vi "Tenscion Analizer.vi"(8 "error in":errorcluster, 11 "Data In":T1) -> (0 "error out":errorcluster, 3 "Data Out":T1)   [LabVIEW 2025]
uses:
  Controls/Wheel_data.ctl
  Controls/Spork plot.ctl
  Controls/Spoke_stats.ctl
  Controls/Spork type.ctl
  Controls/Tension.ctl
  Controls/Tension_Output.ctl
  Controls/Runout.ctl
  Controls/Runout Output.ctl
  Controls/Nippel Turn Direction.ctl
  Controls/Aditional Info.ctl
  <vilib>/Analysis/NI_AALBase.lvlib
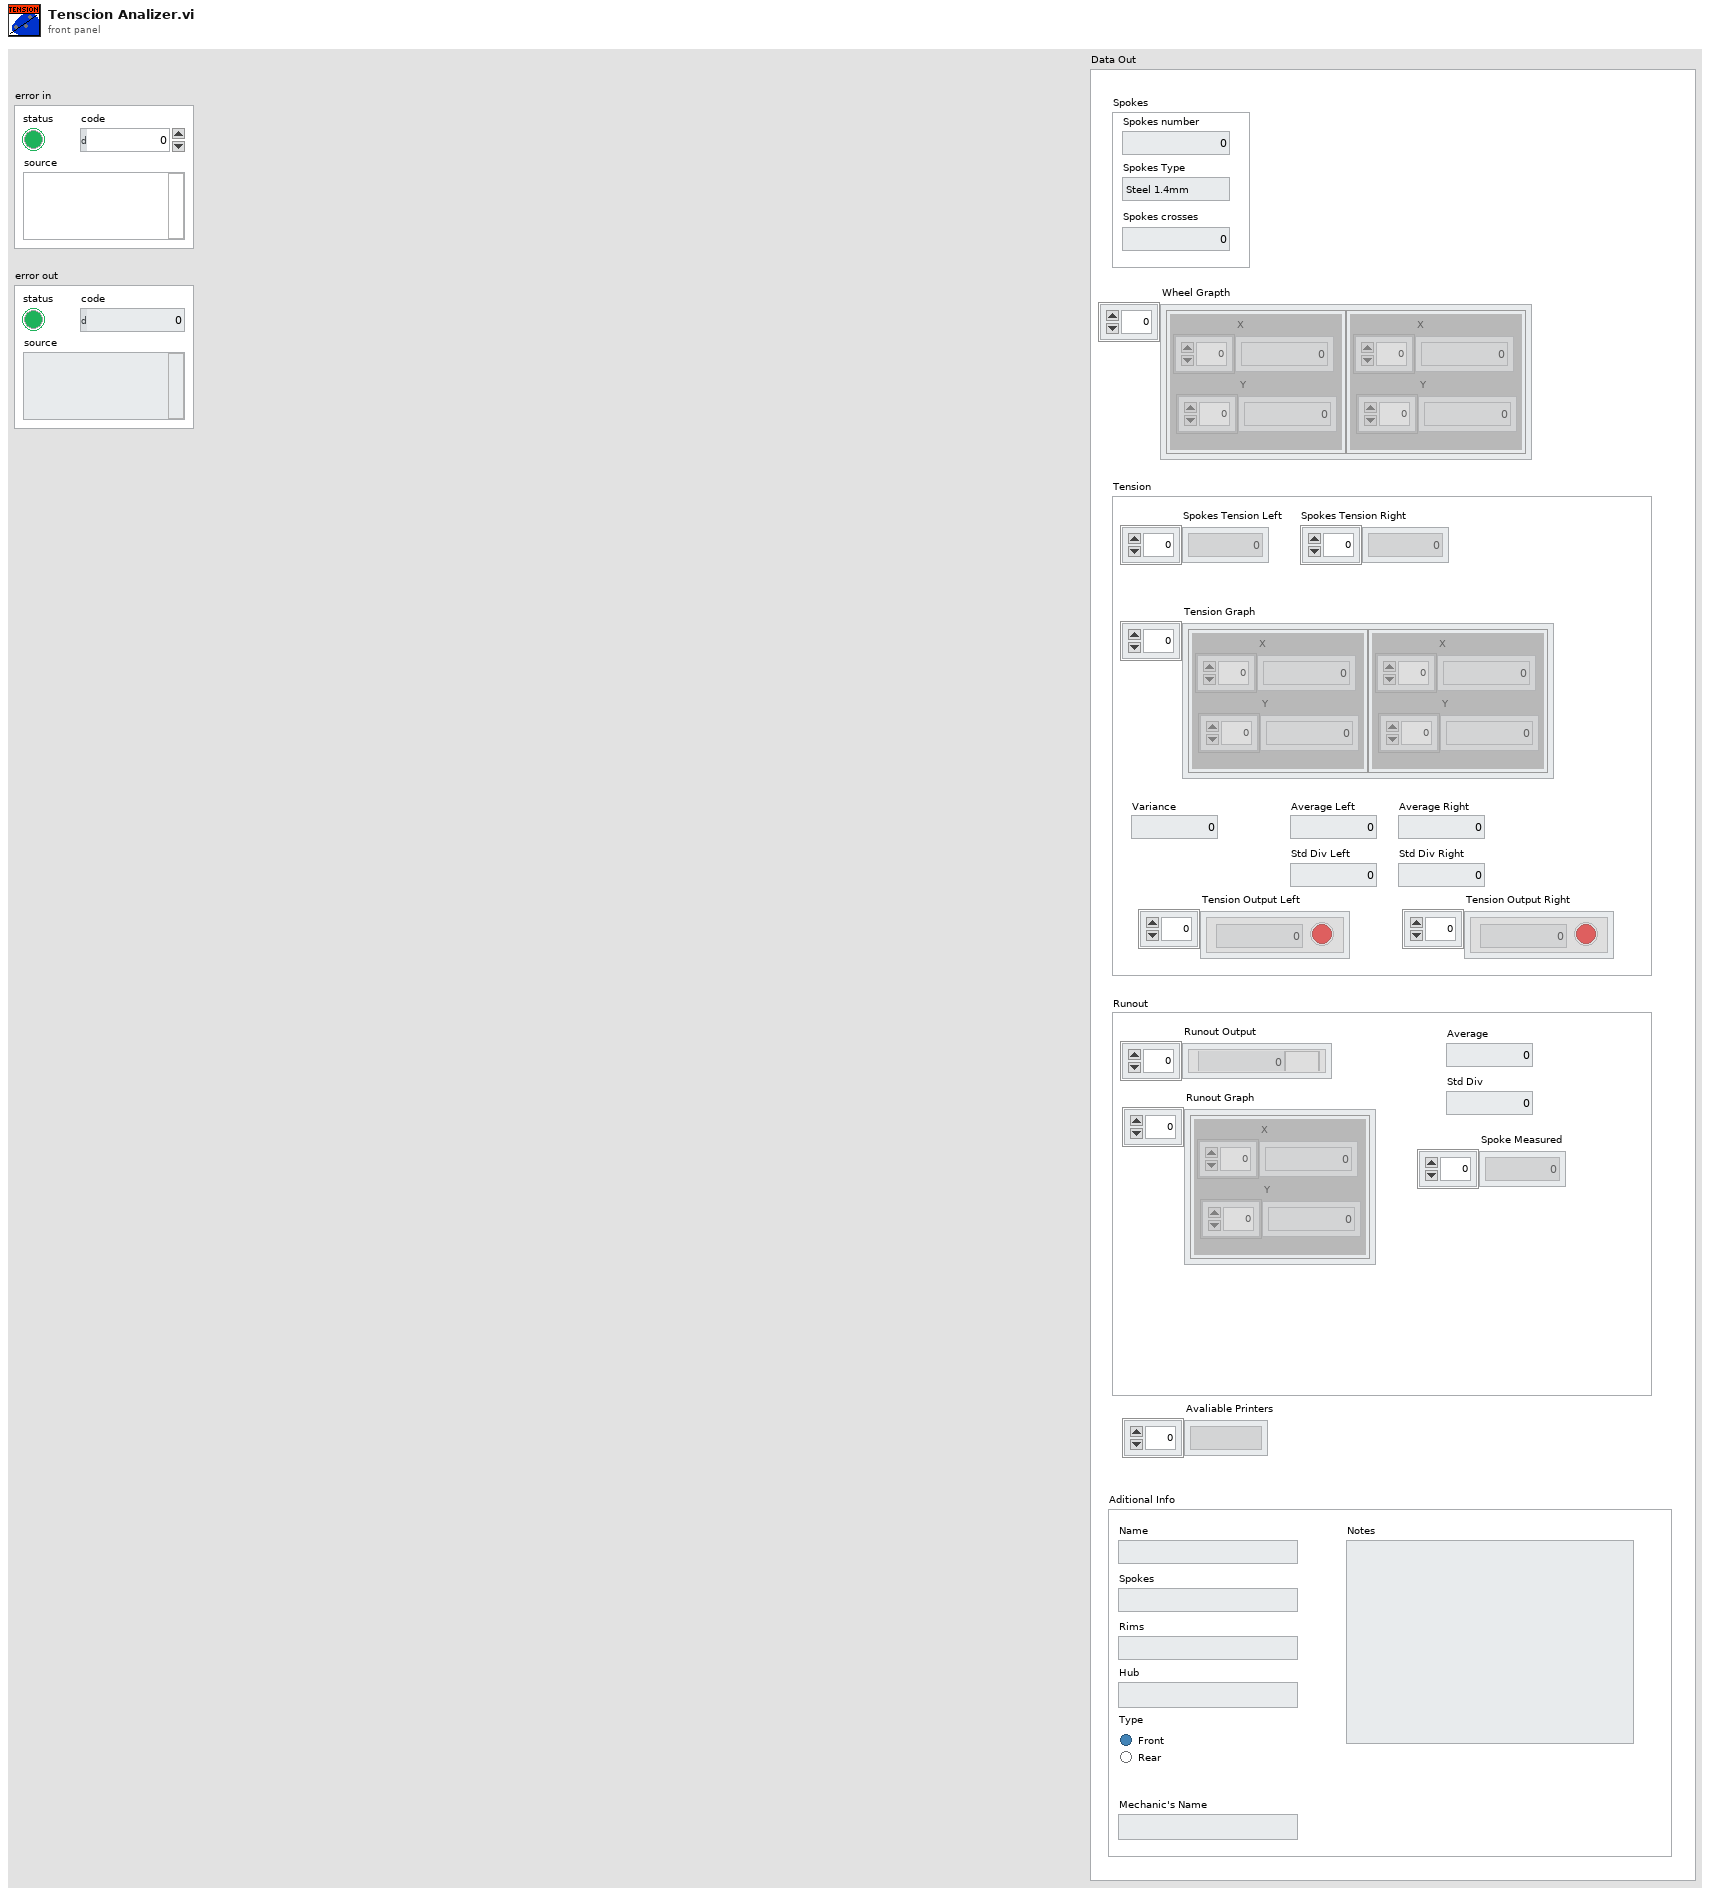
[diagram p1: front panel]
types:
  T1 = typedef "Wheel_data.ctl" = cluster{"Wheel Grapth":T2[], "Spokes":T3, "Tension":T5, "Runout":T7, "Avaliable Printers":string[], "Aditional Info":T10}
  T2 = typedef "Spork plot.ctl" = cluster{"X":dbl[], "Y":dbl[]}
  T3 = typedef "Spoke_stats.ctl" = cluster{"Spokes number":i32, "Spokes crosses":i32, "Spokes Type":T4}
  T4 = typedef "Spork type.ctl" = enum16{"Steel 1.4mm", "Steel 1.5mm", "Steel 1.6mm", "Steel 1.7mm", "Steel 1.8mm", "Steel 2mm", "Steel 2.3mm", "Steel 2.5mm", "Steel 2.6mm", "Aluminum 2.28mm", "Aluminum 2.54mm", "Aluminum 2.8mm", "Aluminum 3.3mm"}
  T5 = typedef "Tension.ctl" = cluster{"Spokes Tension Left":dbl[], "Tension Graph":T2[], "Average Left":dbl, "Variance":dbl, "Std Div Left":dbl, "Average Right":dbl, "Std Div Right":dbl, "Tension Output Left":T6[], "Tension Output Right":T6[], "Spokes Tension Right":dbl[]}
  T6 = typedef "Tension_Output.ctl" = cluster{"Tenction [kgf]":dbl, "Within Limit":bool}
  T7 = typedef "Runout.ctl" = cluster{"Runout Output":T8[], "Runout Graph":T2[], "Average":dbl, "Std Div":dbl, "Spoke Measured":i32[]}
  T8 = typedef "Runout Output.ctl" = cluster{"Value":dbl, "Nippel Direction":T9}
  T9 = typedef "Nippel Turn Direction.ctl" = u16
  T10 = typedef "Aditional Info.ctl" = cluster{"Name":string, "Rims":string, "Hub":string, "Notes":string, "Spokes":string, "Type":enum32{"Item 0", "Item 1"}, "Mechanic's Name":string}
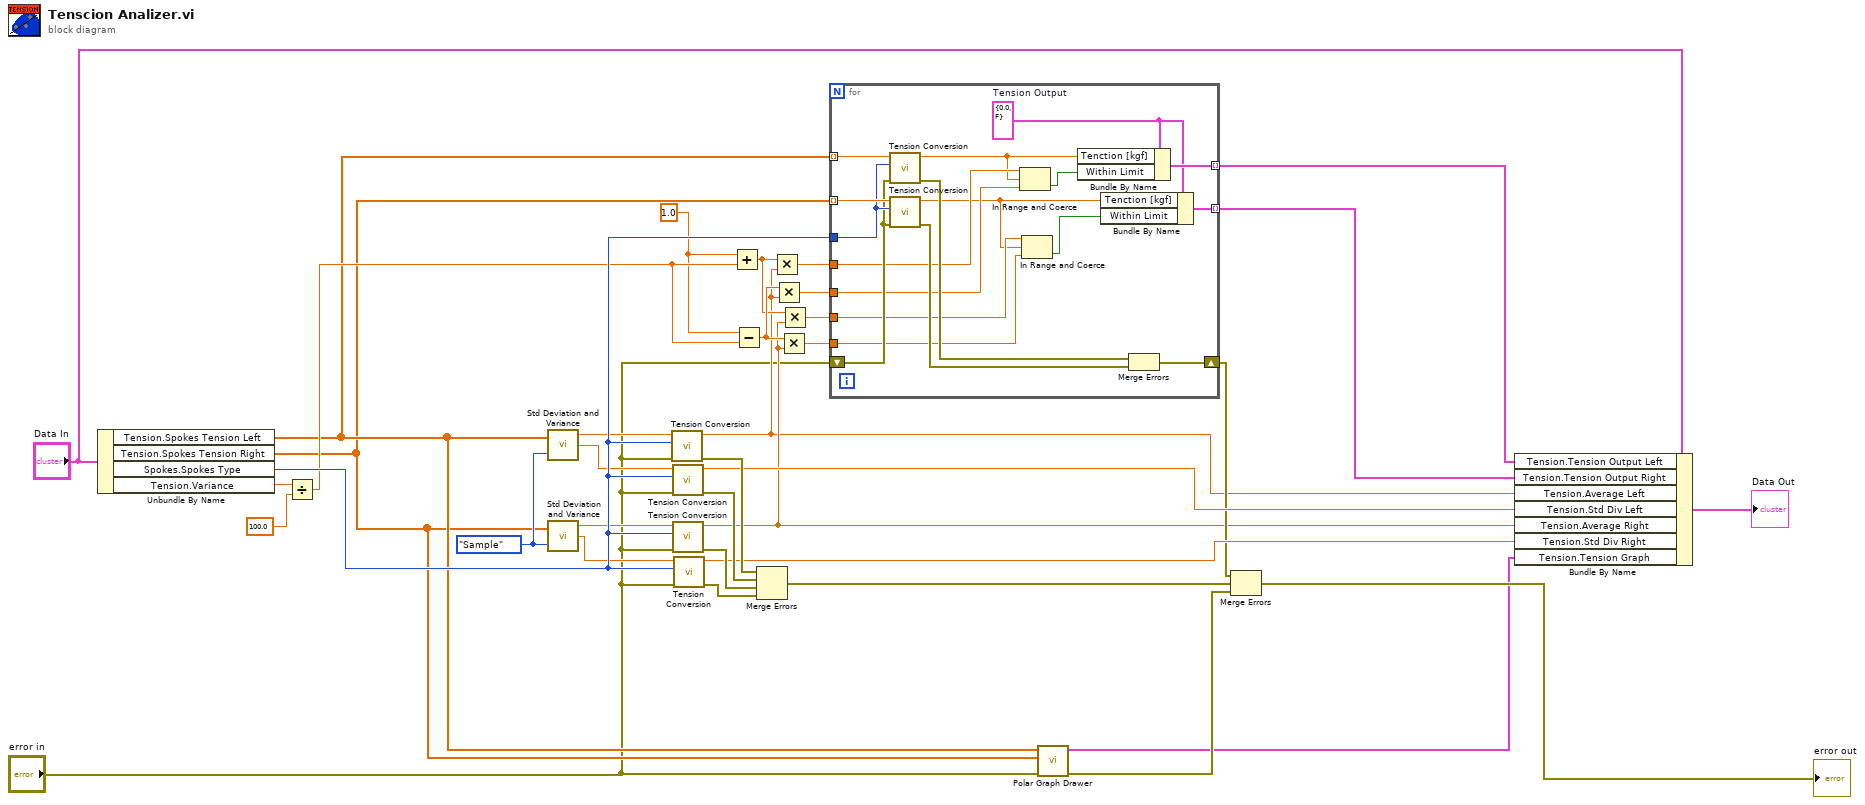
[diagram p0: block diagram]
diagram:
  w22 = 1.0 ("x")
  w7 = enum16{"Sample", "Population"}."Sample" ("Weighting (Sample)")
  n1 = Unbundle By Name("Data In") -> ("Tension.Spokes Tension Left"=w6:dbl[], "Tension.Spokes Tension Right"=w5:dbl[], "Spokes.Spokes Type"=w28:T4, "Tension.Variance"=w25:dbl)
  n2 = Divide(x=w25, y=100.0) -> (x/y=w23:dbl)
  n3 = call <vilib>:"Std Deviation and Variance.vi"("X"=w6, "Weighting (Sample)"=w7) -> ("mean"=w27:dbl, "standard deviation"=w18:dbl)  [unwired: 1 out]
  n4 = call <vilib>:"Std Deviation and Variance.vi"("X"=w5, "Weighting (Sample)"=w7) -> ("mean"=w26:dbl, "standard deviation"=w16:dbl)  [unwired: 1 out]
  n5 = call "Tension Conversion.vi"("error in"="error in", "Spoke Type"=w28, "Tension Input"=w27) -> ("error out"=w31:errorcluster, "Tension [kgf]"=w8:dbl)  [unwired: 6 in, 1 out]
  n6 = call "Tension Conversion.vi"("error in"="error in", "Spoke Type"=w28, "Tension Input"=w18) -> ("error out"=w32:errorcluster, "Tension [kgf]"=w30:dbl)  [unwired: 6 in, 1 out]
  n7 = call "Tension Conversion.vi"("error in"="error in", "Spoke Type"=w28, "Tension Input"=w26) -> ("error out"=w33:errorcluster, "Tension [kgf]"=w9:dbl)  [unwired: 6 in, 1 out]
  n8 = call "Tension Conversion.vi"("error in"="error in", "Spoke Type"=w28, "Tension Input"=w16) -> ("error out"=w34:errorcluster, "Tension [kgf]"=w29:dbl)  [unwired: 6 in, 1 out]
  n9 = Add(x=w22, y=w23) -> (x+y=w15:dbl)
  n10 = Subtract(x=w22, y=w23) -> (x-y=w19:dbl)
  n11 = Merge Errors(w31, w32, w33, w34) -> (w10:errorcluster)
  n12 = Multiply(x=w15, y=w8) -> (x*y=w21:dbl)
  n13 = Multiply(x=w19, y=w8) -> (x*y=w17:dbl)
  n14 = Multiply(x=w19, y=w9) -> (x*y=w20:dbl)
  n15 = Multiply(x=w15, y=w9) -> (x*y=w14:dbl)
  n16 = for {
    tunnel: w6 -> [w53] mode=indexing
    tunnel: w5 -> [w54] mode=indexing
    tunnel: w28 -> [w52]
    shift-right: [w50] -> w11
    shift-left: "error in" -> [w51]
    tunnel: w21 -> [w47]
    tunnel: w20 -> [w44]
    tunnel: w17 -> [w46]
    tunnel: w14 -> [w45]
    tunnel: [w39] -> w13 mode=indexing
    tunnel: [w38] -> w12 mode=indexing
    w37 = T6 {"Tenction [kgf]"=0.0, "Within Limit"=FALSE}  # Tension Output
    n17 = call "Tension Conversion.vi"("error in"=w51, "Spoke Type"=w52, "Tension Input"=w53) -> ("error out"=w48:errorcluster, "Tension [kgf]"=w43:dbl)  [unwired: 6 in, 1 out]
    n18 = call "Tension Conversion.vi"("error in"=w51, "Spoke Type"=w52, "Tension Input"=w54) -> ("error out"=w49:errorcluster, "Tension [kgf]"=w41:dbl)  [unwired: 6 in, 1 out]
    n19 = In Range and Coerce(upper limit=w47, x=w43, lower limit=w46) -> (In Range?=w42:bool)  [unwired: 1 out]
    n20 = In Range and Coerce(upper limit=w45, x=w41, lower limit=w44) -> (In Range?=w40:bool)  [unwired: 1 out]
    n21 = Bundle By Name(cluster=w37, "Tenction [kgf]"=w43, "Within Limit"=w42) -> (w39:T6)
    n22 = Bundle By Name(cluster=w37, "Tenction [kgf]"=w41, "Within Limit"=w40) -> (w38:T6)
    n23 = Merge Errors(w48, w49) -> (w50:errorcluster)
  }
  n24 = call "Polar Graph Drawer.vi"("error in"="error in", "Plot Right"=w5, "Plot Left"=w6) -> ("error out"=w2:errorcluster, "Polar Graph"=w1:cluster{dbl[], dbl[]}[])  [unwired: 7 in]
  n25 = Merge Errors(w11, w10, w2) -> (→"error out":errorcluster)
  n26 = Bundle By Name(cluster="Data In", "Tension.Tension Output Left"=w13, "Tension.Tension Output Right"=w12, "Tension.Average Left"=w8, "Tension.Std Div Left"=w30, "Tension.Average Right"=w9, "Tension.Std Div Right"=w29, "Tension.Tension Graph"=w1) -> (→"Data Out":T1)
